vi "TrigerDelayer_TriggerRate_Set.vi"(8 "error in (no error)":errorcluster, 10 "Trigger Rate":dbl, 11 "VISA Refnum in":refnum<visa-resource-name>) -> (0 "error out":errorcluster, 3 "VISA Refnum out":refnum<visa-resource-name>)   [LabVIEW 2016, in "Trigger Delayer.lvlib"]
uses:
  Trigger Delayer.lvlib
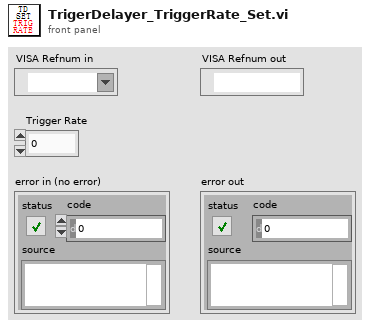
[diagram p1: front panel]
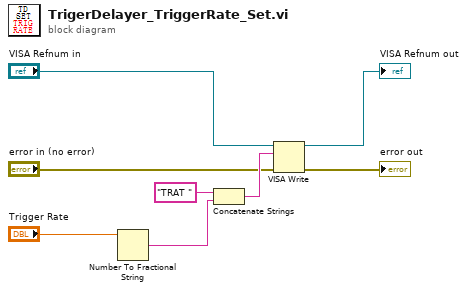
[diagram p0: block diagram]
diagram:
  n1 = Number To Fractional String(number="Trigger Rate") -> (F-format string=w5:string)  [unwired: 3 in]
  n2 = Concatenate Strings("TRAT ", w5) -> (w6:string)
  n3 = VISA Write(VISA resource name="VISA Refnum in", write buffer=w6, error in (no error)="error in (no error)") -> (VISA resource name out=→"VISA Refnum out":refnum<visa-resource-name>, error out=→"error out":errorcluster)  [unwired: 1 out]
